vi "Drive Motor Init.vi"(11 "Error In":errorcluster) -> (2 "Drive Motor Handle":T1, 3 "Error Out":errorcluster)   [LabVIEW 2019]
uses:
  Drive Motor Handle.ctl
  <vilib>/Instr/_visa.llb/VISA Configure Serial Port (Instr).vi
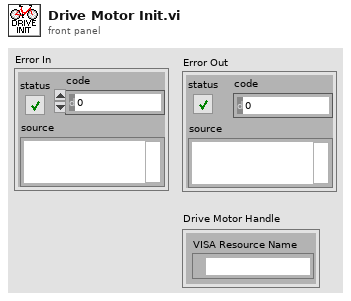
[diagram p1: front panel]
types:
  T1 = typedef "Drive Motor Handle.ctl" = cluster{"VISA Resource Name":refnum<visa-resource-name>}
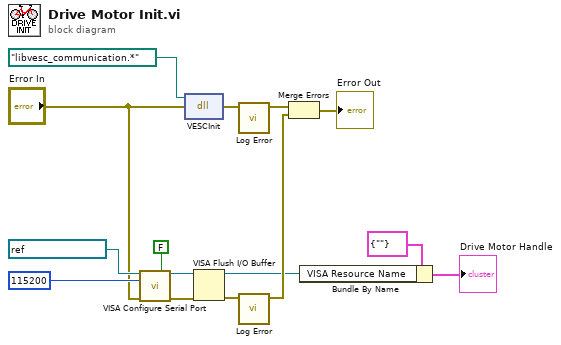
[diagram p0: block diagram]
diagram:
  n1 = call-poly "VISA Configure Serial Port"("VISA resource name"=refnum<visa-resource-name> "ASRL2::INSTR", "Enable Termination\nChar (T)"=FALSE ("Enable Termination\nChar (T)"), "baud rate (9600)"=u32 115200, "error in (no error)"="Error In") -> ("VISA resource name out"=w10:refnum<visa-resource-name>, "error out"=w9:errorcluster)  [unwired: 10 in]
  n2 = dll-call lib="?" fn="VESCInit"(path in=path "libvesc_communication.*", error in="Error In") -> (error out=w14:errorcluster)  [unwired: 2 in, 1 out]
  n3 = VISA Flush I/O Buffer(VISA resource name=w10, error in (no error)=w9) -> (VISA resource name out=w1:refnum<visa-resource-name>, error out=w3:errorcluster)  [unwired: 1 in]
  n4 = call "Log Error.vi"("Error In"=w14) -> ("Error Out"=w5:errorcluster)  [unwired: 10 in]
  n5 = call "Log Error.vi"("Error In"=w3) -> ("Error Out"=w2:errorcluster)  [unwired: 10 in]
  n6 = Merge Errors(w5, w2) -> (→"Error Out":errorcluster)
  n7 = Bundle By Name(cluster=T1 {"VISA Resource Name"=""} ("Drive Motor Handle"), "VISA Resource Name"=w1) -> (→"Drive Motor Handle":T1)
